vi "VISA_Write+Read.vi"(7 "Read?":bool=TRUE, 8 "error in (no error)":errorcluster, 10 "Write Buffer":string, 11 "VISA resource name":refnum<visa-resource-name>) -> (0 "error out":errorcluster, 2 "readout":string, 3 "VISA resource name out":refnum<visa-resource-name>)   [LabVIEW 2012, in "Micos_uic.lvlib"]
doc: "This Utility VI is a wrapper which writes to the instrument and reads the response. This VI is intended to be used as a private VI and altering it could cause several public VI's to operate incorrectly."
uses:
  <instrlib>/Micos_uic/Micos_uic.lvlib
  <vilib>/Utility/error.llb/DialogType.ctl
panel:
  out "appended array":string[](array[string])
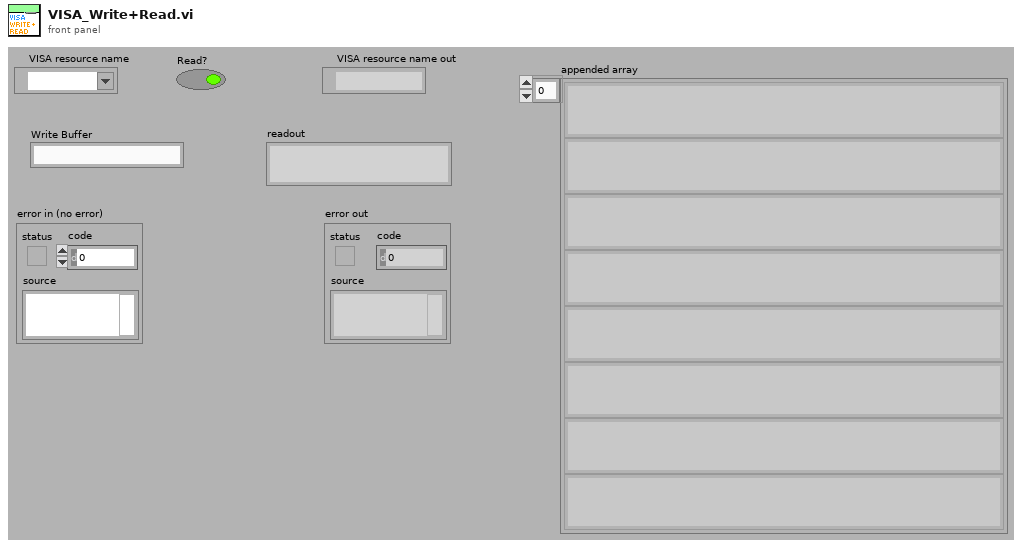
[diagram p1: front panel]
types:
  T1 = typedef "DialogType.ctl" = u16
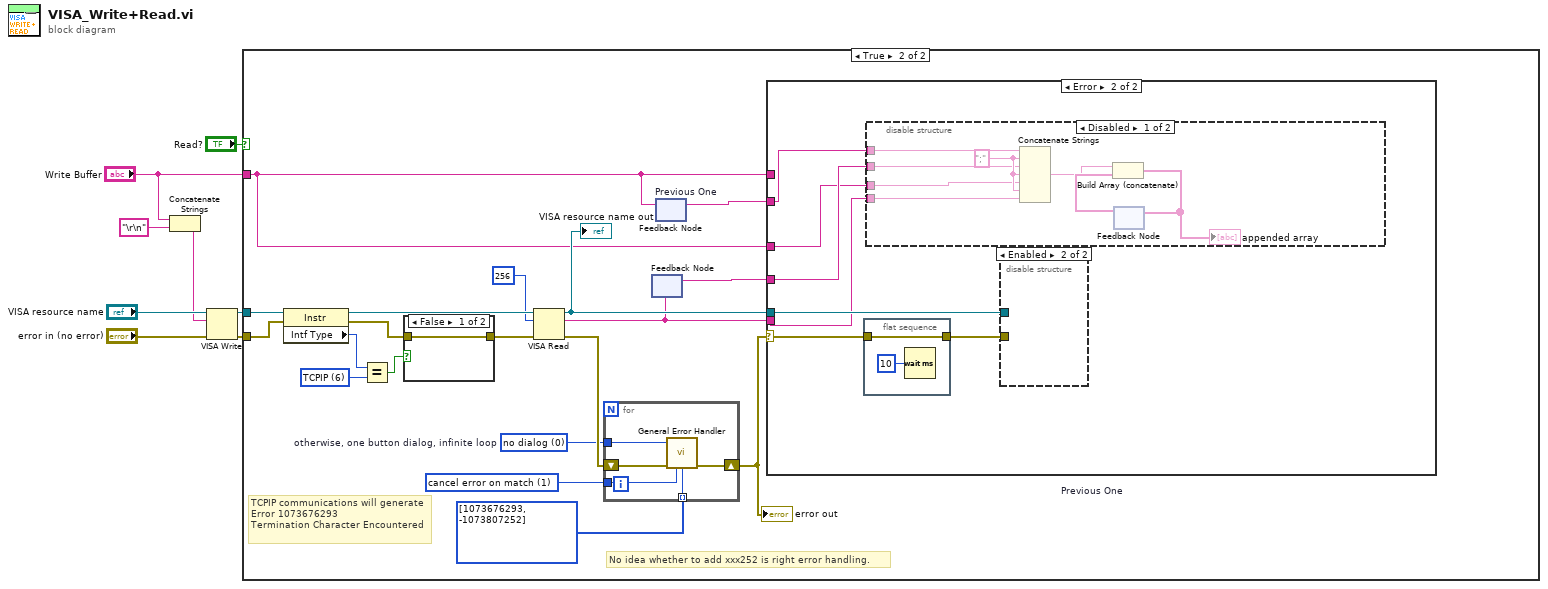
[diagram p0: block diagram]
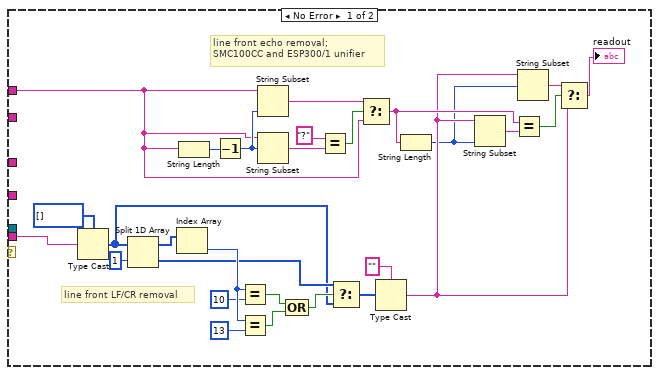
[diagram p3: hidden frame]
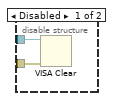
[diagram p5: hidden frame]
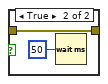
[diagram p6: hidden frame]
diagram:
  n1 = Concatenate Strings("Write Buffer", "\r\n") -> (w1:string)
  n2 = VISA Write(VISA resource name="VISA resource name", write buffer=w1, error in (no error)="error in (no error)") -> (VISA resource name out=w6:refnum<visa-resource-name>, error out=w5:errorcluster)  [unwired: 1 out]
  n3 = case shown="True" "Read?" {
    tunnel: w6 -> [_ w23]
    tunnel: w5 -> [_ w17]
    tunnel: "Write Buffer" -> [_ w12]
    frame False {
    }
    frame True {
      w16 = T1 0 items=["no dialog", "OK message", "continue or stop message", "OK message + warnings", "continue/stop + warnings"]  # otherwise, one button dialog, infinite loop
      w20 = u16 6 items=["GPIB"=1, "VXI"=2, "GPIB-VXI"=3, "Serial"=4, "PXI"=5, "TCPIP"=6, "USB"=7, "FireWire"=9] ("Interface Information:Interface Type")
      w27 = 1 items=["no exception", "cancel error on match", "set error on match"] ("[exception action] (none:0)")
      # "No idea whether to add xxx252 is right error handling."
      # "TCPIP communications will generate\nError 1073676293\nTermination Character Encountered"
      n4 = property class="Instr"(reference=w23, error in=w17) -> (reference out=w22:refnum<visa-resource-name>, error out=w24:errorcluster, "Intf Type"=w19:u16)
      n5 = Equal?(x=w19, y=w20) -> (x = y?=w21:bool)
      n6 = case shown="False" w21 {
        tunnel: [w80 w81] -> w25
        tunnel: w24 -> [w80 w81]
        frame False {
        }
        frame True {
          n7 = Wait (ms)(milliseconds to wait=u32 50) -> ()  [unwired: 1 out]
        }
      }
      n8 = VISA Read(VISA resource name=w22, byte count=u32 256, error in (no error)=w25) -> (VISA resource name out=w14:refnum<visa-resource-name>, read buffer=w11:string, error out=w26:errorcluster)  [unwired: 1 out]
      "VISA resource name out" <- w14
      n9 = for {
        tunnel: w27 -> [w32]
        tunnel: w16 -> [w30]
        shift-right: [w29] -> w15
        shift-left: w26 -> [w31]
        tunnel: i32[] [1073676293, -1073807252] -> [w28] mode=indexing
        n10 = call <vilib>:"General Error Handler.vi"("type of dialog (OK msg:1)"=w30, "error in (no error)"=w31, "[exception action] (none:0)"=w32, "[exception code]"=w28) -> ("error out"=w29:errorcluster)  [unwired: 7 in, 4 out]
      }
      "error out" <- w15
      n11 = feedback #1 "Previous One"() -> (w10:string)  [unwired: 1 in]
      n12 = feedback-in #1(w11) -> ()
      n13 = feedback-in #2(w12) -> ()
      n14 = feedback #2 "Previous One"() -> (w13:string)  [unwired: 1 in]
      n15 = case shown="Error" w15 {
        selector: w15 -> [_ w65]
        tunnel: w11 -> [w35 w61]
        tunnel: w12 -> [w34 _]
        tunnel: w14 -> [_ w67]
        tunnel: w12 -> [_ w62]
        tunnel: w13 -> [_ w64]
        tunnel: w10 -> [_ w63]
        frame No Error {
          # "line front LF/CR removal"
          # "line front echo removal;\nSMC100CC and ESP300/1 unifier"
          n16 = Type Cast(type=u8[] [], x=w35) -> (*(type *) &x=w50:u8[])
          n17 = Split 1D Array(array=w50, index=1) -> (first subarray=w55:u8[], second subarray=w51:u8[])
          n18 = Index Array(array=w55) -> (element=w54:u8)  [unwired: 1 in]
          n19 = String Length(string=w34) -> (length=w44:i32)
          n20 = Decrement(x=w44) -> (x-1=w37:i32)
          n21 = Equal?(x=w54, y=u8 10) -> (x = y?=w59:bool)
          n22 = Equal?(x=w54, y=u8 13) -> (x = y?=w60:bool)
          n23 = String Subset(string=w34, length (rest)=w37) -> (substring=w43:string)  [unwired: 1 in]
          n24 = String Subset(string=w34, offset (0)=w37) -> (substring=w47:string)  [unwired: 1 in]
          n25 = Compound Arithmetic op=OR(w59, w60) -> (w58:bool)
          n26 = Equal?(x="?" ("regular expression"), y=w47) -> (x = y?=w45:bool)
          n27 = Select(t=w51, s=w58, f=w50) -> (s? t:f=w49:u8[])
          n28 = Select(t=w43, s=w45, f=w34) -> (s? t:f=w41:string)
          n29 = Type Cast(type="" ("read buffer"), x=w49) -> (*(type *) &x=w38:string)
          n30 = String Length(string=w41) -> (length=w36:i32)
          n31 = String Subset(string=w38, length (rest)=w36) -> (substring=w42:string)  [unwired: 1 in]
          n32 = Equal?(x=w41, y=w42) -> (x = y?=w40:bool)
          n33 = String Subset(string=w38, offset (0)=w36) -> (substring=w39:string)  [unwired: 1 in]
          n34 = Select(t=w39, s=w40, f=w38) -> (s? t:f=→"readout":string)
        }
        frame Error {
          n35 = flat-sequence {
            tunnel: [w78] -> w66
            tunnel: w65 -> [w78]
            frame #0 {
              n36 = Wait (ms)(milliseconds to wait=u32 10) -> ()  [unwired: 1 out]
            }
          }
          n37 = disable-structure shown="Disabled" {
            disable-tunnel: w64 -> [w73 _]
            disable-tunnel: w63 -> [w70 _]
            disable-tunnel: w62 -> [w69 _]
            disable-tunnel: w61 -> [w68 _]
            frame Disabled {
              w71 = ";" ("string")
              n38 = Concatenate Strings(w73, w71, w70, w71, w69, w71, w68) -> (w74:string)
              n39 = feedback #3() -> (w75:string[])  [unwired: 1 in]
              n40 = Build Array (concatenate)(w74, w75) -> (w72:string[])
              "appended array" <- w72
              n41 = feedback-in #3(w72) -> ()
            }
            frame Enabled {
            }
          }
          n42 = disable-structure shown="Enabled" {
            disable-tunnel: w67 -> [w77 _]
            disable-tunnel: w66 -> [w76 _]
            frame Disabled {
              n43 = VISA Clear(VISA resource name=w77, error in (no error)=w76) -> ()  [unwired: 2 out]
            }
            frame Enabled {
            }
          }
        }
      }
    }
  }
